vi "FieldDisp_Convert_IMAQ_Image_to_Picture.vi"(8 "error in (no error)":errorcluster, 11 "Image In":T1) -> (0 "error out":errorcluster, 3 "new picture":picture)   [LabVIEW 2019, in "Trajectory_Library.lvlib"]
doc: "Internal function -- should not be called directly by users.\n\nComplete documentation TBD."
uses:
  <vilib>/vision/Image Controls.llb/IMAQ Image.ctl
  Trajectory_Library.lvlib
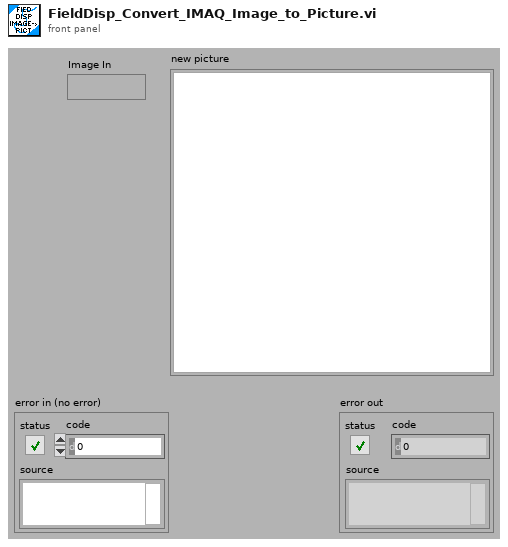
[diagram p1: front panel]
types:
  T1 = typedef "IMAQ Image.ctl" = refnum<image>
  T2 = typedef "imagedata.ctl" = cluster{"image type":i32, "image depth":i32, "image":u8[], "mask":u8[], "colors":u32[], "Rectangle":cluster{"left":i16, "top":i16, "right":i16, "bottom":i16}}
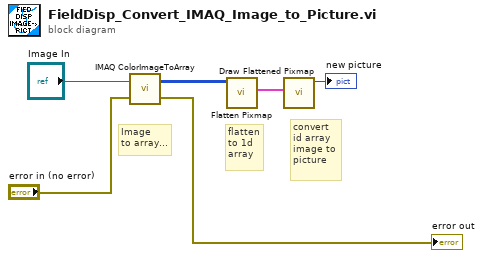
[diagram p0: block diagram]
diagram:
  # "convert\nid array\nimage to\npicture"
  # "flatten\nto 1d \narray"
  # "Image\nto array..."
  n1 = call "IMAQ ColorImageToArray"("Image"="Image In", "error in (no error)"="error in (no error)") -> ("Image Pixels (U32)"=w3:u32[][], "error out"=→"error out":errorcluster)  [unwired: 2 in, 1 out]
  n2 = call <vilib>:"Flatten Pixmap.vi"("24-bit pixmap"=w3) -> ("image data"=w5:T2)  [unwired: 5 in, 5 out]
  n3 = call <vilib>:"Draw Flattened Pixmap.vi"("image data"=w5) -> ("new picture"=→"new picture":picture)  [unwired: 1 in, 7 out]
